vi "terminate.vi"(8 "error in (no error)":errorcluster, 11 "DL090211ImageAssemblerScaffold in":refnum<class "ImageAssemblerDL090211Scaffold.lvclass">) -> (0 "error out":errorcluster, 3 "DL090211ImageAssemblerScaffold out":refnum<class "ImageAssemblerDL090211Scaffold.lvclass">)   [LabVIEW 2010, in "ImageAssemblerDL090211Scaffold.lvclass"]
uses:
  ImageAssemblerDL090211Scaffold.lvclass
  common/classes/Image/Image/Image.lvclass
  GenericImageAssembler/GenericImageAssembler/GenericImageAssembler.lvclass
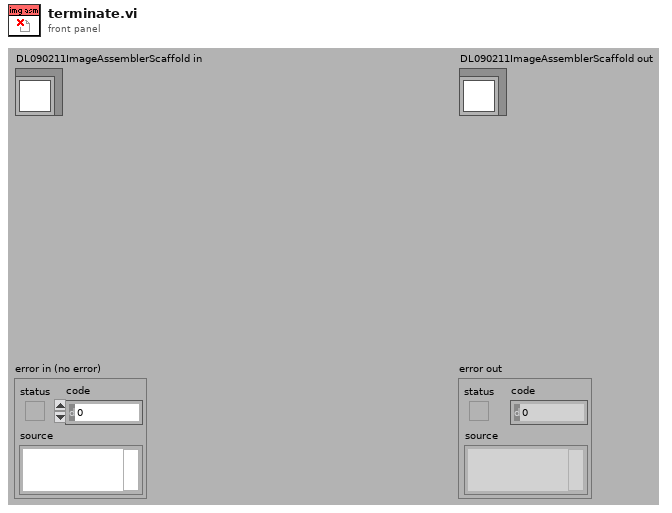
[diagram p1: front panel]
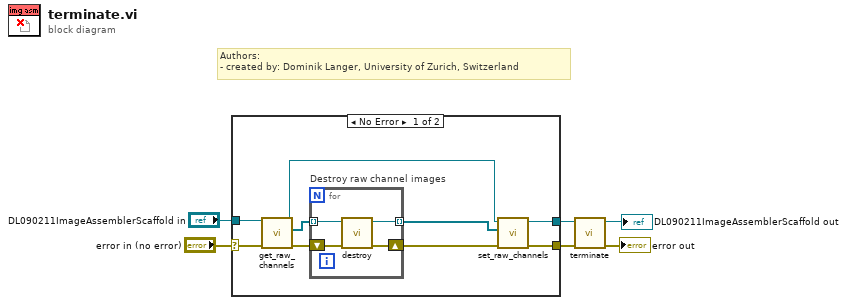
[diagram p0: block diagram]
diagram:
  # "Authors: \n- created by: Dominik Langer, University of Zurich, Switzerland"
  n1 = case shown="No Error" "error in (no error)" {
    selector: "error in (no error)" -> [w14 w21]
    tunnel: [w7 w21] -> w4
    tunnel: [w8 w20] -> w1
    tunnel: "DL090211ImageAssemblerScaffold in" -> [w9 w20]
    frame No Error {
      n2 = call-dynamic "get_raw_channels.vi"("error in (no error)"=w14, "DL090211ImageAssemblerScaffold.lvclass in"=w9) -> ("error out"=w13:errorcluster, "raw channels"=w15:refnum<class "Image.lvclass">[], "DL090211ImageAssemblerScaffold.lvclass out"=w10:refnum<class "ImageAssemblerDL090211Scaffold.lvclass">)  [unwired: 7 out]
      n3 = for "Destroy raw channel images" {
        shift-right: [w17] -> w12
        shift-left: w13 -> [w19]
        tunnel: w15 -> [w18] mode=indexing
        tunnel: [w16] -> w11 mode=indexing
        n4 = call-dynamic "destroy.vi"("error in (no error)"=w19, "Image in"=w18) -> ("error out"=w17:errorcluster, "Image out"=w16:refnum<class "Image.lvclass">)  [unwired: 8 out]
      }
      n5 = call "set_raw_channels.vi"("error in (no error)"=w12, "raw channels"=w11, "DL090211ImageAssemblerScaffold.lvclass in"=w10) -> ("error out"=w7:errorcluster, "DL090211ImageAssemblerScaffold.lvclass out"=w8:refnum<class "ImageAssemblerDL090211Scaffold.lvclass">)  [unwired: 7 out]
    }
    frame Error {
    }
  }
  n6 = call-parent "terminate.vi"("error in (no error)"=w4, "GenericPlugin in"=w1) -> ("error out"=→"error out":errorcluster, "GenericPlugin out"=→"DL090211ImageAssemblerScaffold out":refnum<class "ImageAssemblerDL090211Scaffold.lvclass">)  [unwired: 8 out]
